vi "Remove Stream.vi"(8 "error in (no error)":errorcluster, 10 "Stream":refnum<data-value>, 11 "CameraManager":refnum<data-value>) -> (0 "error out":errorcluster, 3 "CameraManager (duplicate)":refnum<data-value>)   [LabVIEW 2020, in "g_ar_toolkit.capture.lvlib" / "CameraManager.lvclass"]
uses:
  CameraManager.lvclass
  CameraStream/CameraStream.lvclass
  CameraManager.lvclass/CameraManager.ctl
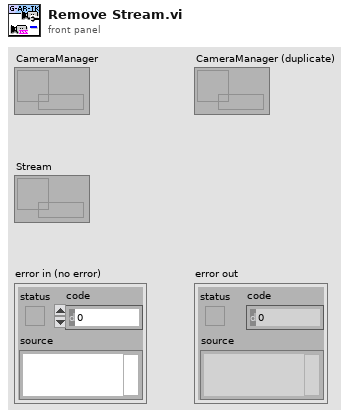
[diagram p1: front panel]
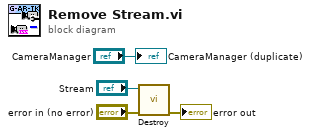
[diagram p0: block diagram]
diagram:
  n1 = call "Destroy.vi"("error in (no error)"="error in (no error)", "Stream"="Stream") -> ("error out"=→"error out":errorcluster)  [unwired: 9 in]
  "CameraManager (duplicate)" <- "CameraManager"
